vi "Save Pretty-Printed XML.vi"(0 "XML Input":string[](array[string]), 1 "XML File Path":path) -> ()   [LabVIEW 2013]
uses:
  <vilib>/Utility/xml.llb/Write to XML File(array).vi
  <vilib>/xml/Load XML File.vi
  <vilib>/xml/NI_XML.lvlib
  <resource>/objmgr/DOMUserDefRef.rc
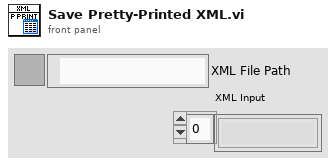
[diagram p1: front panel]
types:
  T1 = enum16{"open", "replace", "create", "open or create", "replace or create", "replace or create with confirmation"}
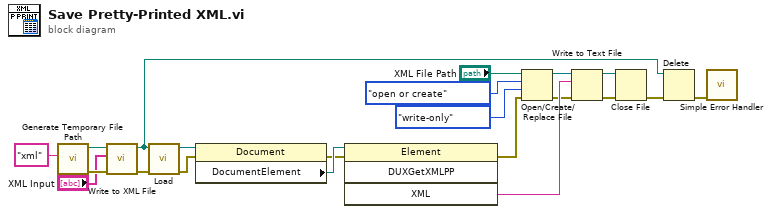
[diagram p0: block diagram]
diagram:
  n1 = call <vilib>:"Generate Temporary File Path.vi"("Temporary File Extension (tmp)"="xml") -> ("error out"=w4:errorcluster, "Unique Temporary File Path"=w3:path)  [unwired: 9 in]
  n2 = call-poly <vilib>:"Write to XML File.vi"("error in (no error)"=w4, "XML Input"="XML Input", "XML File Path"=w3) -> ("error out"=w5:errorcluster, "XML File Path"=w20:path)  [unwired: 6 in, 1 out]
  n3 = call-poly <vilib>:"Load.vi"("path to XML document"=w20, "error in (no error)"=w5) -> ("DOM document out"=w7:refnum<k20>, "error out"=w6:errorcluster)  [unwired: 11 in, 1 out]
  n4 = property class="Document"(reference=w7, error in=w6) -> (error out=w8:errorcluster, "DocumentElement"=w9:refnum<k20>)  [unwired: 1 out]
  n5 = invoke class="Element" method="DUXGetXMLPP"(reference=w9, error in=w8) -> (error out=w18:errorcluster, "XML"=w15:string)  [unwired: 2 in, 2 out]
  n6 = Open/Create/Replace File(file path (use dialog)="XML File Path", error in=w18, operation (0:open)=T1."open or create", access (0:read/write)=enum16{"read/write", "read-only", "write-only"}."write-only") -> (refnum out=w14:refnum<file>, error out=w13:errorcluster)  [unwired: 2 in, 1 out]
  n7 = Write to Text File(file (use dialog)=w14, text=w15, error in=w13) -> (refnum out=w17:refnum<file>, error out=w16:errorcluster)  [unwired: 1 in, 1 out]
  n8 = Close File(refnum=w17, error in=w16) -> (error out=w19:errorcluster)  [unwired: 1 out]
  n9 = Delete(path (use dialog)=w20, error in=w19) -> (error out=w21:errorcluster)  [unwired: 3 in, 2 out]
  n10 = call <vilib>:"Simple Error Handler.vi"("error in (no error)"=w21) -> ()  [unwired: 4 in, 5 out]
